vi "Rohde & Schwarz VNA Preset.vi"(8 "error in (no error)":errorcluster, 11 "VISA Resource Name":refnum<visa-resource-name>) -> (0 "error out":errorcluster, 3 "dup VISA Resource Name":refnum<visa-resource-name>)   [LabVIEW 2011]
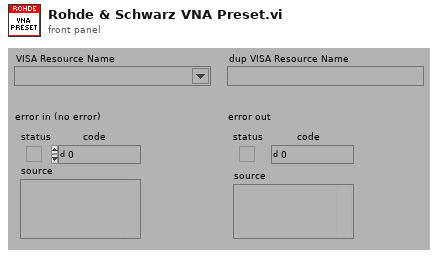
[diagram p1: front panel]
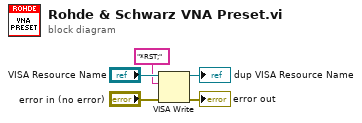
[diagram p0: block diagram]
diagram:
  n1 = VISA Write(VISA resource name="VISA Resource Name", write buffer="*RST;", error in (no error)="error in (no error)") -> (VISA resource name out=→"dup VISA Resource Name":refnum<visa-resource-name>, error out=→"error out":errorcluster)  [unwired: 1 out]
